vi "Drive Encoder.vi"(10 "Reset":bool, 11 "Enum":enum16{"Init", "Run", "End"}(ring)) -> (3 "Encoder Values":T1)   [LabVIEW 2011]
uses:
  TypeDefs/Digital Module 1.ctl
  <vilib>/Rock Robotics/SystemInterfaces/Typedef/FPGA_TypedefDigitalModule.ctl
  <vilib>/Rock Robotics/SystemInterfaces/DIO/FPGA_DIOChannel.ctl
  <vilib>/Rock Robotics/WPI/Encoder/WPI_EncoderType.ctl
  <vilib>/Rock Robotics/WPI/Counter/WPI_CounterDigitalInputToDigitalSource.vi
panel:
  in  "Number Samples to Average":u8=1 min=1 max=128
  in  "Minimum Rate":dbl=20.0
  in  "Decoding Type":T2=enum."4x"
  in  "Digital Module A":T3={"Module"=enum."Digital Module 1", "Left Enc A"=enum."DIO 1", "Left Enc B"=enum."DIO 2", "Right Enc A"=enum."DIO 3", "Right Enc B"=enum."DIO 4", "Outer Sensor"=enum."DIO 5", "Inner Sensor"=enum."DIO 6", "Upper Sensor"=enum."DIO 7", "Shooter Tachometer"=enum."DIO 8", "Unassigned"=enum."DIO 9", "Unassigned"=enum."DIO 10", "Top Conveyer Sensor"=enum."DIO 11", "Arm Upper Limit"=enum."DIO 12", "Arm Lower Limit"=enum."DIO 13", "1510"=enum."DIO 14"}
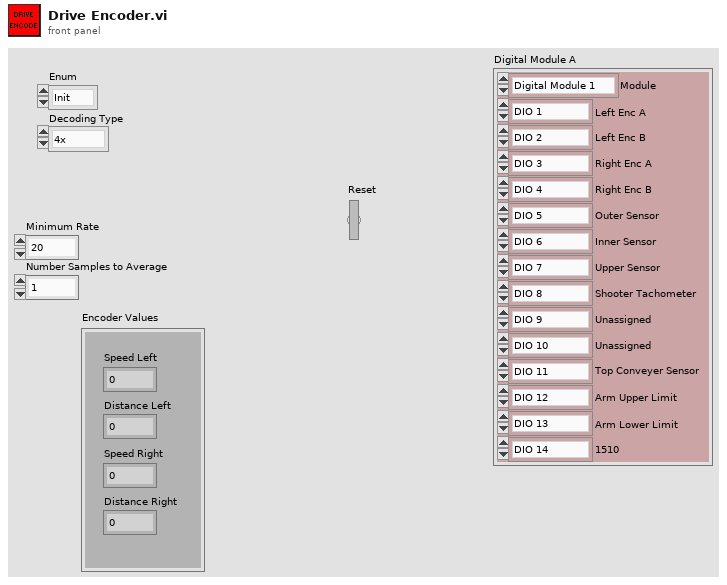
[diagram p1: front panel]
types:
  T1 = cluster{"Speed Right":dbl, "Distance Right":dbl, "Speed Left":dbl, "Distance Left":dbl}
  T2 = typedef "WPI_EncoderType.ctl" = enum16{"1x", "2x", "4x"}
  T3 = typedef "Digital Module 1.ctl" = cluster{"Module":T4, "Left Enc A":T5, "Left Enc B":T5, "Right Enc A":T5, "Right Enc B":T5, "Outer Sensor":T5, "Inner Sensor":T5, "Upper Sensor":T5, "Shooter Tachometer":T5, "Unassigned":T5, "Unassigned":T5, "Top Conveyer Sensor":T5, "Arm Upper Limit":T5, "Arm Lower Limit":T5, "1510":T5}
  T4 = typedef "FPGA_TypedefDigitalModule.ctl" = enum16{"Digital Module 1", "Digital Module 2"}
  T5 = typedef "FPGA_DIOChannel.ctl" = enum8{"DIO 1", "DIO 2", "DIO 3", "DIO 4", "DIO 5", "DIO 6", "DIO 7", "DIO 8", "DIO 9", "DIO 10", "DIO 11", "DIO 12", "DIO 13", "DIO 14", "Invalid"}
  T6 = typedef "WPI_DigitalInputDevRef.ctl" = cluster{"DevStatus":errorcluster, "DIO Channel":T5, "Digital Module":T4}
  T7 = typedef "FPGA_CounterEncoderSourceConvertionLVSourceType.ctl" = cluster{"DevStatus":errorcluster, "AnalogTriggerMode?":bool, "DigitalMode":cluster{"Digital Module":T4, "DIO Channel":T8}, "AnalogTriggerMode":cluster{"AnalogTriggerIndex":T9, "OutputType":T10}}
  T8 = typedef "FPGA_DIODigitalSourceChannel.ctl" = enum8{"DIO 1", "DIO 2", "DIO 3", "DIO 4", "DIO 5", "DIO 6", "DIO 7", "DIO 8", "DIO 9", "DIO 10", "DIO 11", "DIO 12", "DIO 13", "DIO 14", "Disabled"}
  T9 = typedef "FPGA_AnalogTriggerIndex.ctl" = enum8{"Trig 0", "Trig 1", "Trig 2", "Trig 3", "Trig 4", "Trig 5", "Trig 6", "Trig 7", "Invalid"}
  T10 = typedef "FPGA_AnalogTriggerOutType.ctl" = enum16{"InWindow", "TriggerState", "Rising", "Falling"}
  T11 = typedef "WPI_EncoderDevRef.ctl" = cluster{"DevStatus":errorcluster, "EncoderIndex":T12, "CounterIndex":T13, "DistancePerCount":dbl, "Decoding Type":T2}
  T12 = typedef "FPGA_EncoderIdx.ctl" = enum8{"Enc 0", "Enc 1", "Enc 2", "Enc 3", "Invalid"}
  T13 = typedef "FPGA_CounterCtrSystemIndex.ctl" = enum8{"Ctr 0", "Ctr 1", "Ctr 2", "Ctr 3", "Ctr 4", "Ctr 5", "Ctr 6", "Ctr 7", "Invalid"}
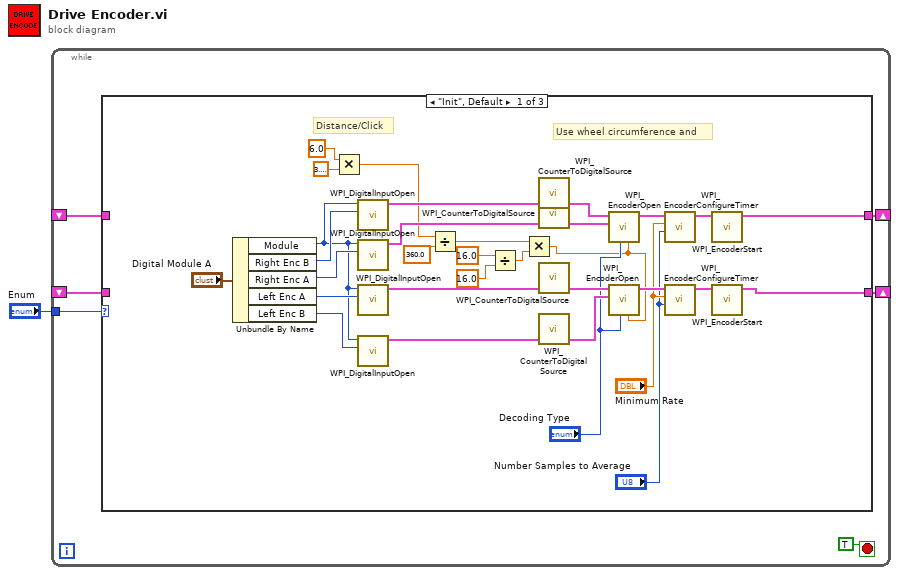
[diagram p0: block diagram]
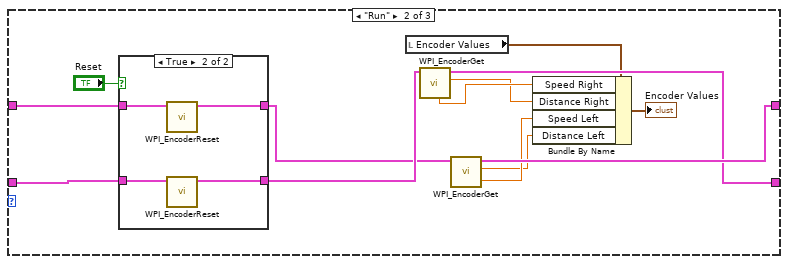
[diagram p2: hidden frame]
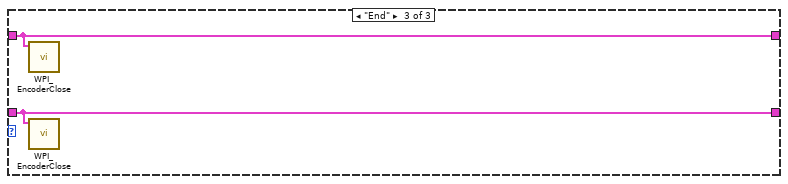
[diagram p4: hidden frame]
diagram:
  n1 = while {
    tunnel: "Enum" -> [w7]
    shift-right: [w5] -> _
    shift-left: _ -> [w4]
    shift-right: [w3] -> _
    shift-left: _ -> [w2]
    stop <- TRUE stop-if-true
    n2 = case shown="\"Init\", Default" w7 {
      tunnel: [w32 w47 w60] -> w5
      tunnel: w4 -> [_ w52 w60]
      tunnel: [w19 w46 w59] -> w3
      tunnel: w2 -> [_ w51 w59]
      frame "Init", Default {
        # "Use wheel circumference and"
        # "Distance/Click"
        n3 = Unbundle By Name("Digital Module A") -> ("Module"=w27:T4, "Right Enc B"=w38:T5, "Right Enc A"=w35:T5, "Left Enc A"=w29:T5, "Left Enc B"=w28:T5)
        n4 = Multiply(x=6.0, y=3.141592653589793) -> (x*y=w14:dbl)
        n5 = call <vilib>:"WPI_DigitalInputOpen.vi"("DIO Channel"=w38, "Digital Module (Module 1)"=w27) -> ("DigitalInputDevRef"=w37:T6)  [unwired: 8 in, 1 out]
        n6 = call <vilib>:"WPI_DigitalInputOpen.vi"("DIO Channel"=w35, "Digital Module (Module 1)"=w27) -> ("DigitalInputDevRef"=w34:T6)  [unwired: 8 in, 1 out]
        n7 = call <vilib>:"WPI_DigitalInputOpen.vi"("DIO Channel"=w29, "Digital Module (Module 1)"=w27) -> ("DigitalInputDevRef"=w26:T6)  [unwired: 8 in, 1 out]
        n8 = call <vilib>:"WPI_DigitalInputOpen.vi"("DIO Channel"=w28, "Digital Module (Module 1)"=w27) -> ("DigitalInputDevRef"=w24:T6)  [unwired: 8 in, 1 out]
        n9 = Divide(x=w14, y=360.0) -> (x/y=w11:dbl)
        n10 = Divide(x=16.0, y=16.0) -> (x/y=w9:dbl)
        n11 = Multiply(x=w11, y=w9) -> (x*y=w12:dbl)
        n12 = call-poly <vilib>:"WPI_CounterToDigitalSource.vi"("DigitalInputDevRef"=w37) -> ("Digital Source"=w36:T7)  [unwired: 6 in]
        n13 = call-poly <vilib>:"WPI_CounterToDigitalSource.vi"("DigitalInputDevRef"=w34) -> ("Digital Source"=w33:T7)  [unwired: 6 in]
        n14 = call-poly <vilib>:"WPI_CounterToDigitalSource.vi"("DigitalInputDevRef"=w26) -> ("Digital Source"=w25:T7)  [unwired: 6 in]
        n15 = call-poly <vilib>:"WPI_CounterToDigitalSource.vi"("DigitalInputDevRef"=w24) -> ("Digital Source"=w23:T7)  [unwired: 6 in]
        n16 = call <vilib>:"WPI_EncoderOpen.vi"("DistancePerCount"=w12, "Decoding Type"="Decoding Type", "BSource"=w33, "ASource"=w36) -> ("EncoderDevRef"=w18:T11)  [unwired: 6 in, 1 out]
        n17 = call <vilib>:"WPI_EncoderOpen.vi"("DistancePerCount"=w12, "Decoding Type"="Decoding Type", "BSource"=w23, "ASource"=w25) -> ("EncoderDevRef"=w21:T11)  [unwired: 6 in, 1 out]
        n18 = call <vilib>:"WPI_EncoderConfigureTimer.vi"("Number Samples to Average"="Number Samples to Average", "Minimum Rate"="Minimum Rate", "EncoderDevRef"=w18) -> ("EncoderDevRef"=w17:T11)  [unwired: 7 in, 1 out]
        n19 = call <vilib>:"WPI_EncoderConfigureTimer.vi"("Number Samples to Average"="Number Samples to Average", "Minimum Rate"="Minimum Rate", "EncoderDevRef"=w21) -> ("EncoderDevRef"=w20:T11)  [unwired: 7 in, 1 out]
        n20 = call <vilib>:"WPI_EncoderStart.vi"("EncoderDevRef"=w17) -> ("EncoderDevRef"=w32:T11)  [unwired: 9 in, 1 out]
        n21 = call <vilib>:"WPI_EncoderStart.vi"("EncoderDevRef"=w20) -> ("EncoderDevRef"=w19:T11)  [unwired: 9 in, 1 out]
      }
      frame "Run" {
        n22 = case shown="True" "Reset" {
          tunnel: w52 -> [w54 w58]
          tunnel: [w54 w57] -> w48
          tunnel: w51 -> [w53 w56]
          tunnel: [w53 w55] -> w49
          frame False {
          }
          frame True {
            n23 = call <vilib>:"WPI_EncoderReset.vi"("EncoderDevRef"=w58) -> ("EncoderDevRef"=w57:T11)  [unwired: 9 in, 1 out]
            n24 = call <vilib>:"WPI_EncoderReset.vi"("EncoderDevRef"=w56) -> ("EncoderDevRef"=w55:T11)  [unwired: 9 in, 1 out]
          }
        }
        n25 = local read "Encoder Values"() -> (w45:T1)
        n26 = call <vilib>:"WPI_EncoderGet.vi"("EncoderDevRef"=w49) -> ("Distance"=w42:dbl, "EncoderDevRef"=w46:T11, "Rate"=w43:dbl)  [unwired: 5 in, 3 out]
        n27 = call <vilib>:"WPI_EncoderGet.vi"("EncoderDevRef"=w48) -> ("Distance"=w40:dbl, "EncoderDevRef"=w47:T11, "Rate"=w41:dbl)  [unwired: 5 in, 3 out]
        n28 = Bundle By Name(cluster=w45, "Speed Right"=w43, "Distance Right"=w42, "Speed Left"=w41, "Distance Left"=w40) -> (→"Encoder Values":T1)
      }
      frame "End" {
        n29 = call <vilib>:"WPI_EncoderClose.vi"("EncoderDevRef"=w60) -> ()  [unwired: 10 in, 1 out]
        n30 = call <vilib>:"WPI_EncoderClose.vi"("EncoderDevRef"=w59) -> ()  [unwired: 10 in, 1 out]
      }
    }
  }
